vi "MPU6050 Read Data.vi"(8 "error in (no error)":errorcluster, 9 "Start Address":u8, 10 "Data Length":u32, 11 "I2C Ref In":T1={"myRIO Reference"={"myRIO Model"=enum."Unknown", "myRIO Hardware Reference"={"Generic FPGA Reference"=refnum, "Allow multiple opens"=FALSE}}, "I2C Channels Enum"=enum."Not Connected", "I2C Configuration"={"I2C Transfer Rate"=enum."Fast mode (400 kbps)"}}) -> (0 "error out":errorcluster, 2 "Data read":u8[](array[numeric]))   [LabVIEW 2018]
uses:
  <vilib>/myRIO/Instrument Drivers/Onboard IO/I2C/typedefs/I2C Reference.ctl
  <vilib>/myRIO/Common/Instrument Driver Framework/Utilities/typedefs/myRIO Generic Hardware Reference.ctl
  <vilib>/myRIO/Common/Instrument Driver Framework/Utilities/typedefs/Hardware Version Enum.ctl
  <vilib>/myRIO/Common/Instrument Driver Framework/Utilities/typedefs/myRIO v1.0 Reference.ctl
  <vilib>/myRIO/Common/Instrument Driver Framework/Utilities/typedefs/Generic FPGA Reference.ctl
  <vilib>/myRIO/Common/Instrument Driver Framework/myRIO v1.0/I2C/typedefs/I2C Channels Enum.ctl
  <vilib>/myRIO/Instrument Drivers/Onboard IO/I2C/typedefs/I2C Configuration.ctl
  <vilib>/myRIO/Instrument Drivers/Onboard IO/I2C/typedefs/I2C Transfer Rate.ctl
  MPU6050 Private class data.vi
  <vilib>/Utility/error.llb/Error Cluster From Error Code.vi
  <vilib>/myRIO/Common/Instrument Driver Framework/myRIO v1.0/I2C/vis/myRIO v1.0 Write I2C.vi
  <vilib>/myRIO/Common/Instrument Driver Framework/myRIO v1.0/I2C/vis/myRIO v1.0 Read I2C.vi
  <vilib>/myRIO/Instrument Drivers/Onboard IO/I2C/I2C.lvlib
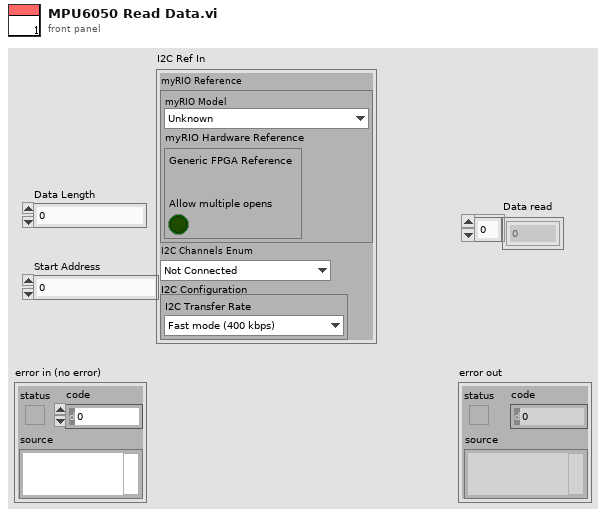
[diagram p1: front panel]
types:
  T1 = typedef "I2C.lvlib/I2C Reference.ctl" = cluster{"myRIO Reference":T2, "I2C Channels Enum":T6, "I2C Configuration":T7}
  T2 = typedef "myRIO Generic Hardware Reference.ctl" = cluster{"myRIO Model":T3, "myRIO Hardware Reference":T4}
  T3 = typedef "Hardware Version Enum.ctl" = enum16{"Unknown", "myRIO-1900", "myRIO-1950", "roboRIO", "NI ELVIS RIO CM", "ELVIS III"}
  T4 = typedef "myRIO v1.0 Reference.ctl" = cluster{"Generic FPGA Reference":T5, "Allow multiple opens":bool}
  T5 = typedef "Generic FPGA Reference.ctl" = refnum<k20>
  T6 = typedef "I2C Channels Enum.ctl" = enum16{"Not Connected", "A/I2C", "B/I2C", "I2C/I2C"}
  T7 = typedef "I2C.lvlib/I2C Configuration.ctl" = cluster{"I2C Transfer Rate":T8}
  T8 = typedef "I2C.lvlib/I2C Transfer Rate.ctl" = enum16{"Standard mode (100 kbps)", "Fast mode (400 kbps)"}
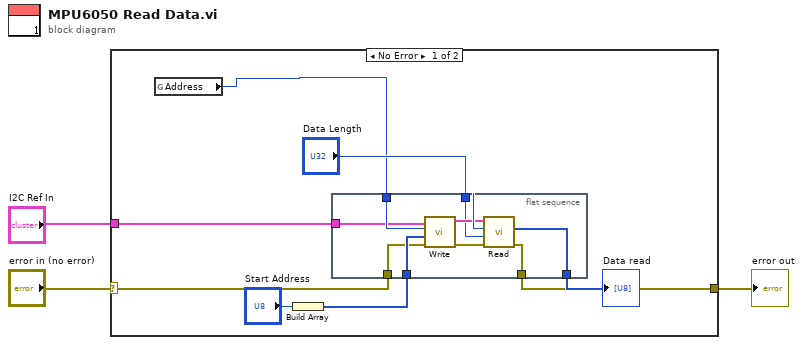
[diagram p0: block diagram]
diagram:
  n1 = case shown="No Error" "error in (no error)" {
    selector: "error in (no error)" -> [w7 w21]
    tunnel: [w6 w21] -> w2
    tunnel: "I2C Ref In" -> [w5 _]
    frame No Error {
      n2 = global read "MPU6050 Private class data.vi" "Address"() -> (w4:u8)
      n3 = Build Array("Start Address") -> (w10:u8[])
      n4 = flat-sequence {
        tunnel: w4 -> [w20]
        tunnel: w10 -> [w18]
        tunnel: "Data Length" -> [w17]
        tunnel: [w16] -> w8
        tunnel: w7 -> [w15]
        tunnel: [w13] -> w6
        tunnel: w5 -> [w12]
        frame #0 {
          n5 = call <vilib>:"Write.vi"("error in (no error)"=w15, "Bytes to Write"=w18, "Slave Address (7-bit)"=w20, "I2C Ref In"=w12) -> ("error out"=w14:errorcluster, "I2C Ref Out"=w19:T1)  [unwired: 6 in]
          n6 = call <vilib>:"Read.vi"("error in (no error)"=w14, "Byte Count"=w17, "Slave Address (7-bit)"=w20, "I2C Ref In"=w19) -> ("error out"=w13:errorcluster, "Bytes Read"=w16:u8[])  [unwired: 4 in, 1 out]
        }
      }
      "Data read" <- w8
    }
    frame Error {
    }
  }
  "error out" <- w2
